vi "Safe Move.vi"(8 "error in (no error)":errorcluster, 11 "Gantry Class in":refnum<class "Gantry Class.lvclass">) -> (0 "error out":errorcluster, 3 "Gantry Class out":refnum<class "Gantry Class.lvclass">)   [LabVIEW 2011, in "Gantry Class.lvclass"]
uses:
  Gantry Class.lvclass
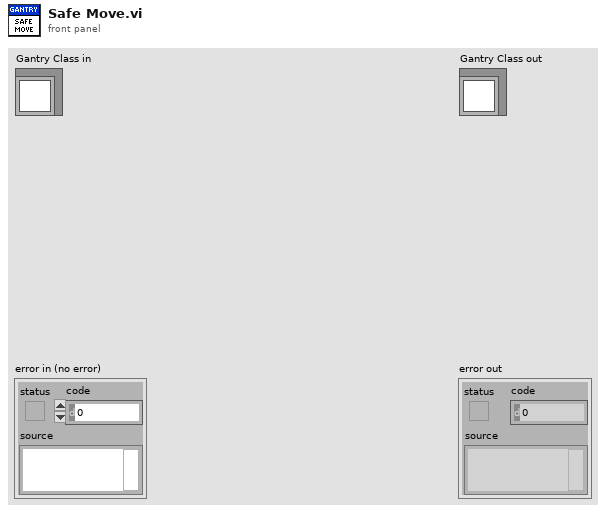
[diagram p1: front panel]
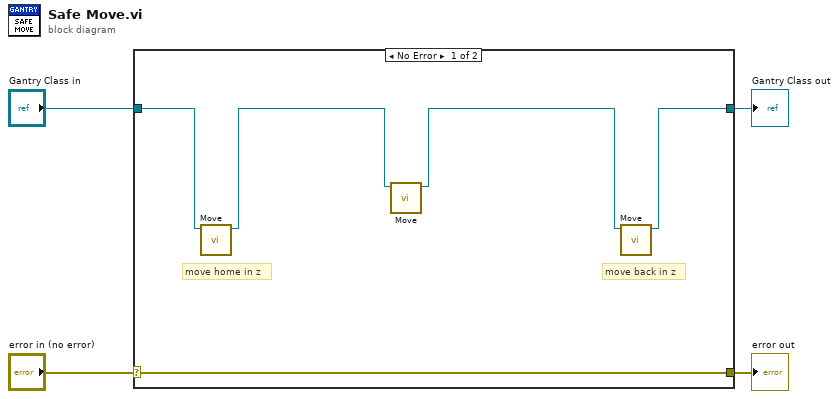
[diagram p0: block diagram]
diagram:
  n1 = case shown="No Error" "error in (no error)" {
    selector: "error in (no error)" -> [w9 w11]
    tunnel: [w9 w11] -> w3
    tunnel: [w5 w10] -> w1
    tunnel: "Gantry Class in" -> [w8 w10]
    frame No Error {
      # "move back in z"
      # "move home in z"
      n2 = call "Move.vi"("Gantry Class in"=w8) -> ("Gantry Class out"=w7:refnum<class "Gantry Class.lvclass">)  [unwired: 9 in, 1 out]
      n3 = call "Move.vi"("Gantry Class in"=w7) -> ("Gantry Class out"=w6:refnum<class "Gantry Class.lvclass">)  [unwired: 9 in, 1 out]
      n4 = call "Move.vi"("Gantry Class in"=w6) -> ("Gantry Class out"=w5:refnum<class "Gantry Class.lvclass">)  [unwired: 9 in, 1 out]
    }
    frame Error {
    }
  }
  "error out" <- w3
  "Gantry Class out" <- w1
